vi "Edit Header.vi"(8 "Error In":errorcluster, 10 "channel name(s)":string[](array[string]), 11 "Table Ref In":refnum<vi>) -> (0 "Error Out":errorcluster, 3 "Table Ref Out":refnum<vi>)   [LabVIEW 2019, in "Table Tools.lvlib"]
doc: "Update Table headers."
uses:
  Table Tools.lvlib
  <vilib>/Utility/miscctls.llb/LVRowAndColumnUnsignedTypeDef.ctl
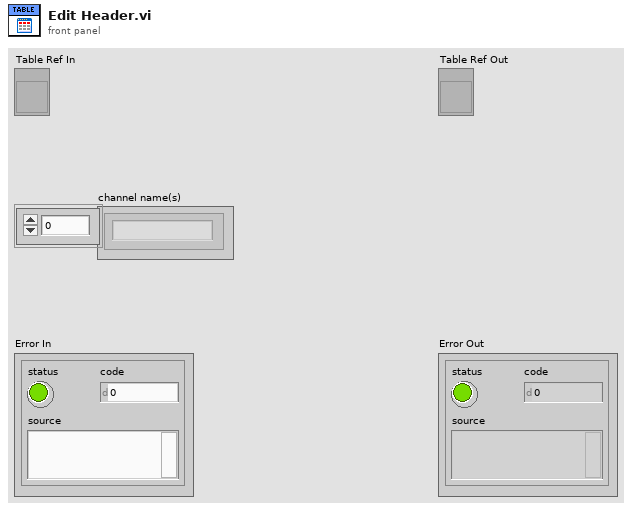
[diagram p1: front panel]
types:
  T1 = typedef "LVRowAndColumnUnsignedTypeDef.ctl" = cluster{"Row":u32, "Column":u32}
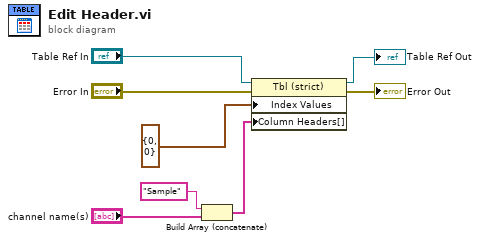
[diagram p0: block diagram]
diagram:
  n1 = Build Array (concatenate)("Sample", "channel name(s)") -> (w7:string[])
  n2 = property on="Property Node" class="Tbl (strict)"(reference="Table Ref In", error in="Error In", "Index Values"=T1 {"Row"=0, "Column"=0}, "Column Headers[]"=w7) -> (reference out=→"Table Ref Out":refnum<vi>, error out=→"Error Out":errorcluster)
